vi "Close caller's caller.vi"(5 "error in (no error)":errorcluster) -> (0 "error out":errorcluster, 2 "call chain":string[](array[string]), 3 "vi reference":refnum<vi>)   [LabVIEW 2016]
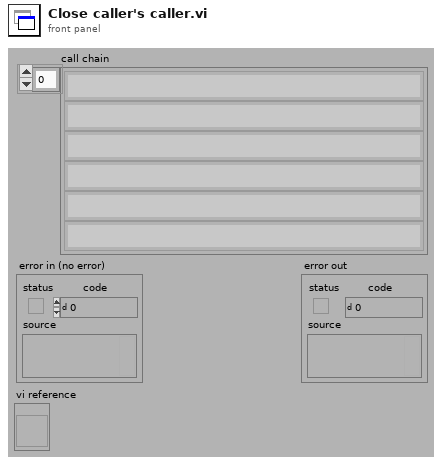
[diagram p1: front panel]
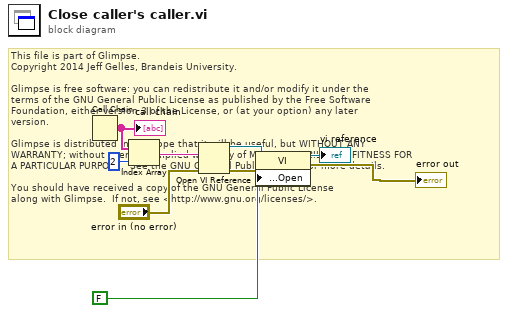
[diagram p0: block diagram]
diagram:
  # "This file is part of Glimpse. \nCopyright 2014 Jeff Gelles, Brandeis University.    \n\nGlimpse is free software: you can redistribute it and/or modify it under the \nterms of the GNU General Public License as published by the Free Software \nFoundation, either version 3 of the License, or (at your option) any later \nversion.\n\nGlimpse is distributed in the hope that it will be useful, but WITHOUT ANY \nWARRANTY; without even the implied warranty of MERCHANTABILITY or FITNESS FOR \nA PARTICULAR PURPOSE.  See the GNU General Public License for more details.\n\nYou should have received a copy of the GNU General Public License\nalong with Glimpse.  If not, see <http://www.gnu.org/licenses/>."
  n1 = Call Chain() -> (call chain=w9:string[])
  "call chain" <- w9
  n2 = Index Array(array=w9, index=2 ("Index")) -> (element=w7:string)
  n3 = Open VI Reference(vi path=w7, error in (no error)="error in (no error)") -> (vi reference=w6:refnum<vi>, error out=w5:errorcluster)  [unwired: 4 out]
  n4 = property class="VI"(reference=w6, error in=w5, "Front Panel Window:Open"=FALSE) -> (reference out=→"vi reference":refnum<vi>, error out=→"error out":errorcluster)
